vi "RIO_DecideCase.vi"(2 "i":i32, 3 "string":string="z=2+3*(x+y)") -> (0 "symbol":string, 1 "case":string)   [LabVIEW 2012]
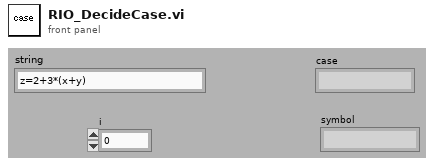
[diagram p1: front panel]
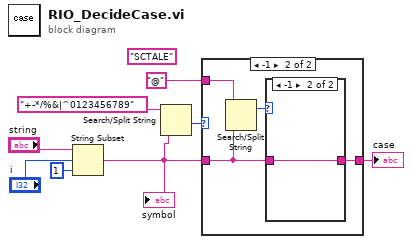
[diagram p0: block diagram]
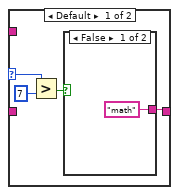
[diagram p2: hidden frame]
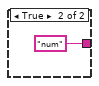
[diagram p3: hidden frame]
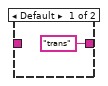
[diagram p4: hidden frame]
diagram:
  (unwired) "SCTALE" ("String")
  n1 = String Subset(string="string", offset (0)="i", length (rest)=1 ("length (rest)")) -> (substring=w3:string)
  "symbol" <- w3
  n2 = Search/Split String(string="+-*/%&|^0123456789" ("String"), search string/char (-)=w3) -> (offset of match=w1:i32)  [unwired: 1 in, 2 out]
  n3 = case shown="-1" w1 {
    selector: w1 -> [w12 _]
    tunnel: [w9 w15] -> w7
    tunnel: w3 -> [_ w16]
    tunnel: "@" ("String") -> [_ w18]
    frame Default {
      n4 = Greater?(x=w12, y=7) -> (0:w10:bool)
      n5 = case shown="False" w10 {
        tunnel: ["math" ("String") "num" ("String")] -> w9
        frame False {
        }
        frame True {
        }
      }
    }
    frame -1 {
      n6 = Search/Split String(string=w18, search string/char (-)=w16) -> (offset of match=w17:i32)  [unwired: 1 in, 2 out]
      n7 = case shown="-1" w17 {
        tunnel: w16 -> [_ w20]
        tunnel: ["trans" ("string") w20] -> w15
        frame Default {
        }
        frame -1 {
        }
      }
    }
  }
  "case" <- w7
